vi "2ndStrikerPositionSkill.vi"(5 "Position":dbl[](array[numeric]), 7 "Time Elapsed?":bool=TRUE, 8 "error in (no error)":errorcluster, 9 "Game in":refnum<class "Game.lvclass">, 10 "Robot":refnum<class "Robot.lvclass">, 11 "2ndStrikerPositionSkill in":refnum<class "2ndStrikerPositionSkill.lvclass">) -> (0 "error out":errorcluster, 2 "2nd Striker Position":dbl[](array[numeric]), 3 "2ndStrikerPositionSkill out":refnum<class "2ndStrikerPositionSkill.lvclass">)   [LabVIEW 2018, in "2ndStrikerPositionSkill.lvclass"]
uses:
  2ndStrikerPositionSkill.lvclass
  Robot_class/Robot.lvclass
  C:/Users/Ronaldo/Desktop/Phoenix GIT/SSL_AI/Object_class/Object.lvclass
  Game_class/Game.lvclass
  Game_class/Game.lvclass/Game.ctl
  Referee_class/Referee.lvclass/Referee.ctl
  Team_class/Team.lvclass/Team.ctl
  Robot_class/Robot.lvclass/Robot.ctl
  Robot_class/roles.ctl
  Object_class/Object.lvclass/Object.ctl
  Utilities_class/Utilities.lvclass
  Object_class/Read x.vi
  Object_class/Read y.vi
  Robot_class/Read id.vi
  0c1a9825-39b9-4625-b9cc-4c6421953776.vi
  Team_class/Read RobotRef.vi
  7c6c6052-d6fd-4101-b52e-e5b07ba4cc6c.vi
  Referee_class/Read enemy_goalie_id.vi
  Game_class/Read EnemyRef.vi
  Game_class/Read AllyRef.vi
  Game_class/Read BallRef.vi
  Game_class/Read FieldRef.vi
  Game_class/Read Referee.vi
  Game_class/Read OffensiveTeam.vi
  <vilib>/Array/Sort 2D Array - Pop Stack.vi
  <vilib>/Array/Sort 2D Array - Push Stack.vi
  Ally_class/Ally.lvclass
  C:/Users/Ronaldo/Desktop/Phoenix GIT/SSL_AI/Team_class/Team.lvclass
  Enemy_class/Enemy.lvclass
  Ball_class/Ball.lvclass
  Field_class/Field.lvclass
  Referee_class/Referee.lvclass
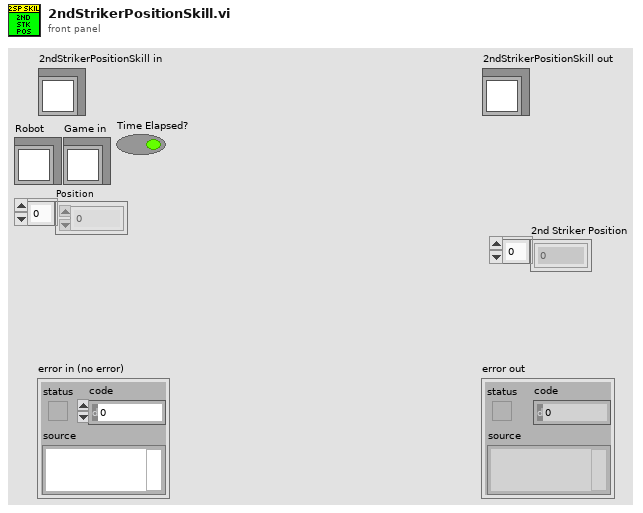
[diagram p1: front panel]
types:
  T1 = typedef "roles.ctl" = enum16{"PenaltyDefense", "PreparePassReceiver", "PassObserver", "Timeout", "Goto", "ZigZag", "None", "BallOutOfField", "DefenderArea", "Duelist", "AttackerStop", "FollowAttacker", "KeeperRole", "KickPenalty", "AttackerAimGoal", "AttackerBlock", "Marker", "Halt", "Shoot", "PassKicker", "PassReceiver", "TestRole", "PenaltyAttacker"}
  T2 = cluster{dbl[][], dbl, "Numeric":dbl, "Numeric":dbl}
  T3 = cluster{dbl[][], dbl, "Numeric":dbl, "Numeric":dbl, "I":dbl[]}
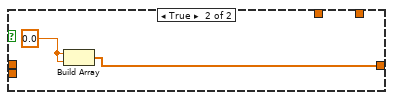
[diagram p3: hidden frame]
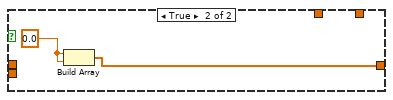
[diagram p4: hidden frame]
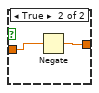
[diagram p5: hidden frame]
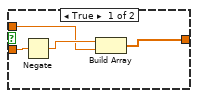
[diagram p9: hidden frame]
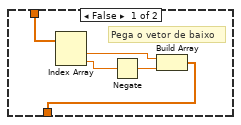
[diagram p10: hidden frame]
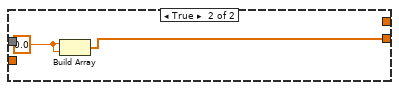
[diagram p12: hidden frame]
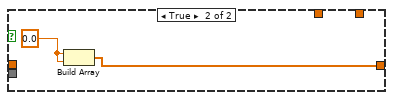
[diagram p13: hidden frame]
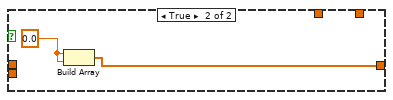
[diagram p17: hidden frame]
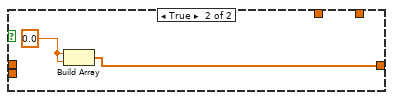
[diagram p18: hidden frame]
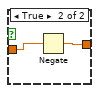
[diagram p19: hidden frame]
diagram:
  n1 = property class="Game"(reference="Game in") -> ("EnemyRef"=w7:refnum<class "Enemy.lvclass">, "AllyRef"=w4:refnum<class "Ally.lvclass">, "BallRef"=w5:refnum<class "Ball.lvclass">, "FieldRef"=w11:refnum<class "Field.lvclass">, "Referee"=w2:refnum<class "Referee.lvclass">, "OffensiveTeam"=w1:refnum<class "Ally.lvclass">)  [unwired: 1 in, 2 out]
  n2 = case shown="No Error" "error in (no error)" {
    selector: "error in (no error)" -> [w30 w734]
    tunnel: [w30 w734] -> w13
    tunnel: [w31 w733] -> w14
    tunnel: "2ndStrikerPositionSkill in" -> [w31 w733]
    tunnel: "Robot" -> [_ _]
    tunnel: w11 -> [w26 _]
    tunnel: w5 -> [_ _]
    tunnel: w7 -> [_ _]
    tunnel: w4 -> [_ _]
    tunnel: "Game in" -> [_ _]
    tunnel: "Time Elapsed?" -> [_ _]
    tunnel: "Position" -> [w29 _]
    tunnel: w7 -> [w25 _]
    tunnel: [w24 _] -> w6
    tunnel: w5 -> [w22 _]
    tunnel: "Robot" -> [w21 _]
    tunnel: w2 -> [w20 _]
    tunnel: w1 -> [w16 _]
    frame No Error {
      # "Verifica se y do 1st str é >= 0"
      n3 = property class="Referee"(reference=w20) -> ("enemy_goalie_id"=w19:i32)  [unwired: 1 in, 2 out]
      n4 = Index Array(array=w29) -> (element #2=w28:dbl)  [unwired: 2 in, 1 out]
      n5 = property class="Ally"(reference=w16) -> ("RobotRef"=w18:refnum<class "Robot.lvclass">[])  [unwired: 1 in, 2 out]
      n6 = Greater Or Equal?(x=w28, y=0.0 ("element")) -> (x >= y?=w23:bool)
      n7 = feedback-in #1(w18) -> ()
      n8 = feedback #1() -> (w17:refnum<class "Robot.lvclass">[])  [unwired: 1 in]
      n9 = case shown="True" w23 {
        tunnel: w26 -> [w137 w489]
        tunnel: w25 -> [w133 w485]
        tunnel: [w122 w474] -> w24
        tunnel: w22 -> [w126 w478]
        tunnel: w21 -> [w108 w460]
        tunnel: w19 -> [w119 w471]
        tunnel: w17 -> [w111 w463]
        frame True {
          w33 = refnum<class "Utilities.lvclass"> refnum ("Utilities in")
          w34 = refnum<class "Utilities.lvclass"> refnum ("Utilities in")
          w99 = refnum<class "Utilities.lvclass"> refnum ("Utilities in")
          (unwired) cluster{dbl[][], dbl, dbl, "y":dbl} {[], 0.0, 0.0, "y"=0.0}
          # "Novo Gap"
          # "Pegar o maior y, faz o mesmo, depois ve qual o maior gap desses 2"
          # "Angulo theta"
          # "Novo Gap"
          # "Pega o vetor de baixo"
          # "Pegar esse menor y, fazer o gap dele com o vetor de baixo e adicionar ao cluster"
          # "O menor y vai ser sempre menor que esse numero"
          # "Aqui entra o cluster"
          # "Tem que pegar os robos que estão nas extremidades, e ver o gap deles com os vetores das extremidades"
          # "Retorna o incentro aqui"
          # "Fazer outro for pra ver se o gap é o maior"
          # "Usar o primeiro elemento como inicial ao inves do zero -> evita erros"
          # "Se todos os robos adversários estão dentro do triangulo, passa as extremidades como robôs"
          # "(Field_length^2 + Field_width^2)^(1/2) / 4"
          # "Ver se a distancia do str é proxima da\ndo 2nd str"
          # "Achar a posição do striker"
          # "Ver se o 2nd striker ta perto do str"
          # "Se o robo esta a uma distância de 200mm da reta bola-gol"
          # "Fazer um if else caso o robo esteja muito proximo da reta do centro do gol ate a bola"
          # "Acha o incentro do triangulo"
          # "O if else evita que divida numero por zero\nSe o modulo do vetor for nulo, ele retorna o (0,0)"
          # "Soma com o vetor (L/2 , 0) pra achar os pontos que os vetores intersectam a reta"
          # "normaliza o vetor e multiplica por A"
          # "a = L/2 (senO/sen(O + O1))"
          # "Transforma os vetores em unitarios"
          # "Verifica quais robos estão na regiao delimitada"
          # "Calcula o ângulo fi (entre o eixo X e o ponto (L/3 , -h/2 -> no caso do triangulo em baixo)"
          # "pega o triangulo de baixo"
          n10 = property class="Enemy"(reference=w133) -> ("RobotRef"=w120:refnum<class "Robot.lvclass">[])  [unwired: 1 in, 2 out]
          n11 = call-dynamic "DeleteRobotByID.vi"("id"=w119, "RobotRef"=w120, "Utilities in"=refnum<class "Utilities.lvclass"> refnum) -> ("RobotRef out"=w118:refnum<class "Robot.lvclass">[])  [unwired: 6 in, 2 out]
          n12 = property class="Field"(reference=w137) -> ("field_length"=w101:i32, "field_width"=w102:i32)  [unwired: 1 in, 2 out]
          n13 = Divide(x=w101, y=6) -> (x/y=w116:dbl)
          n14 = Multiply(x=w116, y=1) -> (x*y=w114:dbl)
          n15 = Divide(x=w101, y=2) -> (x/y=w65:dbl)
          n16 = Divide(x=w102, y=2) -> (x/y=w129:dbl)
          n17 = Build Array(w65, 0.0 ("element")) -> (w44:dbl[])
          n18 = for {
            tunnel: w118 -> [w383] mode=indexing
            tunnel: w44 -> [w377]
            tunnel: [w381] -> w93 mode=indexing if=w372
            # "Só vai considerar os robos dentro da regiao, com y<0 e x>0 (depois do meio campo)"
            # "Trabalhar com os angulos em modulo, e ver se o y é menor que zero"
            n19 = property class="Robot"(reference=w383) -> ("x"=w373:dbl, "y"=w378:dbl, "id"=w371:i32)  [unwired: 1 in, 2 out]
            n20 = Build Array(w373, w378) -> (w382:dbl[])
            n21 = Subtract(x=w382, y=w377) -> (x-y=w380:dbl[])
            n22 = Negate(x=w377) -> (-x=w376:dbl[])
            n23 = call "AngleBetween2Vectors.vi"("Array 1"=w376, "Array 2"=w380, "Utilities in"=refnum<class "Utilities.lvclass"> refnum) -> ("Numeric"=w375:dbl)  [unwired: 6 in, 2 out]
            n24 = Build Array (concatenate)(w380, w375, w371) -> (w381:dbl[])
            n25 = Greater?(x=w373, y=0.0) -> (0:w372:bool)
          }
          n26 = Build Array(w114, w129) -> (w113:dbl[])
          n27 = Build Array(w102, w101) -> (w100:i32[])
          n28 = Subtract(x=w113, y=w44) -> (x-y=w43:dbl[])
          n29 = Negate(x=w44) -> (-x=w127:dbl[])
          n30 = call-dynamic "Module.vi"("2D vector"=w100, "Utilities in"=w99) -> ("Modulo"=w98:dbl)  [unwired: 7 in, 2 out]
          n31 = call "AngleBetween2Vectors.vi"("Array 1"=w127, "Array 2"=w43, "Utilities in"=w99) -> ("Numeric"=w87:dbl)  [unwired: 6 in, 2 out]
          n32 = for {
            tunnel: w93 -> [w195] mode=indexing
            tunnel: w87 -> [w193]
            shift-right: [w190] -> w94
            shift-left: TRUE -> [w191]
            (unwired) TRUE
            n33 = Index Array(array=w195) -> (element #3=w194:dbl)  [unwired: 3 in, 2 out]
            n34 = Less Or Equal?(x=w194, y=w193) -> (x <= y?=w192:bool)
            n35 = And(x=w191, y=w192) -> (x .and. y?=w190:bool)
          }
          n36 = case shown="True" w94 {
            tunnel: w93 -> [w196 w208]
            tunnel: [w196 w207] -> w92
            tunnel: w43 -> [_ w205]
            tunnel: w87 -> [_ w199]
            frame False {
            }
            frame True {
              # "Adiciona os vetores das extremidades"
              n37 = Index Array(array=w205) -> (element #1=w204:dbl, element #2=w203:dbl)  [unwired: 2 in]
              n38 = Build Array (concatenate)(w205, w199, 10) -> (w201:dbl[])
              n39 = Negate(x=w203) -> (-x=w202:dbl)
              n40 = Build Array(w204, w202) -> (w200:dbl[])
              n41 = Build Array (concatenate)(w200, w199, 11) -> (w197:dbl[])
              n42 = Insert Into Array(array=w208, new element #1=w201, new element #2=w197) -> (w207:dbl[][])  [unwired: 2 in]
            }
          }
          n43 = call "Sort 2D Array.vim"("index"=1, "dimension to index (column)"=enum16{"column", "row"}."column", "2D array"=w92) -> ("sorted 2D array"=w91:dbl[][])  [unwired: 7 in, 1 out]
          n44 = Index Array(array=w91) -> (element #1=w90:dbl[])  [unwired: 4 in, 1 out]
          n45 = Index Array(array=w90) -> (element #1=w89:dbl, element #2=w82:dbl, element #3=w80:dbl)  [unwired: 4 in, 1 out]
          n46 = Less?(x=w82, y=0.0) -> (x < y?=w81:bool)
          n47 = case shown="False" w81 {
            tunnel: [w179 w181] -> w79
            tunnel: w80 -> [w179 w180]
            frame False {
            }
            frame True {
              n48 = Negate(x=w180) -> (-x=w181:dbl)
            }
          }
          n49 = Build Array(w89, w82) -> (w88:dbl[])
          n50 = for {
            tunnel: w91 -> [w367] mode=indexing
            shift-right: [w354] -> _
            shift-left: w79 -> [w361]
            shift-right: [w365] -> _
            shift-left: w88 -> [w364]
            tunnel: [w362] -> w128 mode=indexing
            # "Pega o modulo pro caso do 0 e de um angulo neg"
            # "Se o y é negativo, faz o angulo ser negativo\npra quando fazer a difrença de um positivo com um neg\nele somar"
            # "Faz a diferença entre os angulos pra achar os gaps"
            n51 = Index Array(array=w367) -> (element #1=w366:dbl, element #2=w356:dbl, element #3=w355:dbl)  [unwired: 3 in]
            n52 = Less?(x=w356, y=0.0) -> (x < y?=w358:bool)
            n53 = case shown="True" w358 {
              tunnel: w355 -> [w368 w370]
              tunnel: [w368 w369] -> w354
              frame False {
              }
              frame True {
                n54 = Negate(x=w370) -> (-x=w369:dbl)
              }
            }
            n55 = Subtract(x=w354, y=w361) -> (x-y=w360:dbl)
            n56 = Absolute Value(x=w360) -> (abs(x)=w359:dbl)
            n57 = Build Array(w366, w356) -> (w365:dbl[])
            n58 = Build Array(w365, w364) -> (w363:dbl[][])
            n59 = Bundle(w363, w359, "Numeric"=w354, "Numeric"=w361) -> (w362:T2)  [unwired: 1 in]
          }
          n60 = for {
            tunnel: w128 -> [w277] mode=indexing
            tunnel: w87 -> [w276]
            tunnel: w44 -> [w295]
            tunnel: w113 -> [w294]
            tunnel: w65 -> [w290]
            tunnel: w44 -> [w283]
            tunnel: w44 -> [w280]
            tunnel: [w255] -> w112
            tunnel: w44 -> [w258]
            tunnel: w44 -> [w274]
            tunnel: w43 -> [w257]
            tunnel: w87 -> [w256]
            tunnel: [w254] -> w56 mode=indexing if=w245
            tunnel: [w250] -> w52
            w255 = refnum<class "Utilities.lvclass"> refnum ("Utilities in")
            w299 = refnum<class "Utilities.lvclass"> refnum ("Utilities in")
            # "Só vai passar aqueles que a bissetriz ta dentro do traingulo"
            # "E o gap é diferente de zeo\npra poder tirar o primeiro elemento"
            # "Se der false, tem que calcular o incentro novo, e o gap novo"
            # "no novo cluster vai ter tudo do antigo, mais o incentro"
            # "Se o incentro esta dentro do triangulo\npassa o incentro certo"
            # "Angulo theta"
            # "Retorna o gap e os vetores que formam o gap"
            # "Ve qual o maior gap"
            n61 = Unbundle(w277) -> (w265:dbl[][], w249:dbl, "Numeric"=w262:dbl, "Numeric"=w261:dbl)
            n62 = Unbundle(w277) -> (w302:dbl[][], "Numeric"=w269:dbl, "Numeric"=w271:dbl)  [unwired: 1 out]
            n63 = Absolute Value(x=w271) -> (abs(x)=w270:dbl)
            n64 = Absolute Value(x=w269) -> (abs(x)=w268:dbl)
            n65 = Index Array(array=w302) -> (element #1=w301:dbl[], element #2=w300:dbl[])  [unwired: 4 in]
            n66 = call-dynamic "Module.vi"("2D vector"=w300, "Utilities in"=w299) -> ("Modulo"=w297:dbl)  [unwired: 7 in, 2 out]
            n67 = call-dynamic "Module.vi"("2D vector"=w301, "Utilities in"=w299) -> ("Modulo"=w298:dbl)  [unwired: 7 in, 2 out]
            n68 = call "AngleBetween2Vectors.vi"("Array 1"=w295, "Array 2"=w294, "Utilities in"=refnum<class "Utilities.lvclass"> refnum) -> ("Numeric"=w250:dbl)  [unwired: 6 in, 2 out]
            n69 = Equal?(x=w298, y=0) -> (x = y?=w285:bool)
            n70 = Add(x=w250, y=w270) -> (x+y=w291:dbl)
            n71 = Add(x=w250, y=w268) -> (x+y=w292:dbl)
            n72 = Sine(x=w250) -> (sin(x)=w289:dbl)
            n73 = Sine(x=w292) -> (sin(x)=w287:dbl)
            n74 = Sine(x=w291) -> (sin(x)=w286:dbl)
            n75 = Equal?(x=w297, y=0) -> (x = y?=w281:bool)
            n76 = Multiply(x=w289, y=w290) -> (x*y=w288:dbl)
            n77 = Divide(x=w288, y=w287) -> (x/y=w284:dbl)
            n78 = case shown="False" w285 {
              tunnel: w301 -> [w351 _]
              tunnel: w298 -> [w350 _]
              tunnel: w284 -> [w349 _]
              tunnel: w283 -> [w346 _]
              tunnel: [w345 w352] -> w278
              frame False {
                n79 = Divide(x=w351, y=w350) -> (x/y=w348:dbl[])
                n80 = Multiply(x=w348, y=w349) -> (x*y=w347:dbl[])
                n81 = Add(x=w346, y=w347) -> (x+y=w345:dbl[])
              }
              frame True {
                w353 = 0.0
                n82 = Build Array(w353, w353) -> (w352:dbl[])
              }
            }
            n83 = Divide(x=w288, y=w286) -> (x/y=w253:dbl)
            n84 = case shown="False" w281 {
              tunnel: w300 -> [w342 _]
              tunnel: w297 -> [w336 _]
              tunnel: w253 -> [w341 _]
              tunnel: w280 -> [w337 _]
              tunnel: [w338 w343] -> w279
              tunnel: [w337 _] -> w252
              tunnel: [w336 _] -> w251
              frame False {
                n85 = Divide(x=w342, y=w336) -> (x/y=w340:dbl[])
                n86 = Multiply(x=w340, y=w341) -> (x*y=w339:dbl[])
                n87 = Add(x=w337, y=w339) -> (x+y=w338:dbl[])
              }
              frame True {
                w344 = 0.0
                n88 = Build Array(w344, w344) -> (w343:dbl[])
              }
            }
            n89 = call "IncenterTriangle.vi"("C"=w279, "B"=w278, "A"=w258, "Utilities in"=w255) -> ("I"=w267:dbl[])  [unwired: 5 in, 2 out]
            n90 = Subtract(x=w267, y=w274) -> (x-y=w275:dbl[])
            n91 = Negate(x=w274) -> (-x=w273:dbl[])
            n92 = call "AngleBetween2Vectors.vi"("Array 1"=w273, "Array 2"=w275, "Utilities in"=w255) -> ("Numeric"=w272:dbl)  [unwired: 6 in, 2 out]
            n93 = Equal?(x=0.0, y=w249) -> (x = y?=w247:bool)
            n94 = Less Or Equal?(x=w272, y=w276) -> (x <= y?=w245:bool)
            n95 = Or(x=w245, y=w247) -> (x .or. y?=w246:bool)
            n96 = case shown="False" w246 {
              tunnel: w267 -> [_ w335]
              tunnel: [w319 w335] -> w266
              tunnel: w265 -> [w324 w334]
              tunnel: [w317 w334] -> w264
              tunnel: w249 -> [_ w333]
              tunnel: [w313 w333] -> w263
              tunnel: w262 -> [_ w332]
              tunnel: w261 -> [w315 w331]
              tunnel: [w316 w332] -> w260
              tunnel: [w315 w331] -> w259
              tunnel: w258 -> [w323 _]
              tunnel: w257 -> [w320 _]
              tunnel: w256 -> [w316 _]
              tunnel: w255 -> [w312 _]
              tunnel: w253 -> [w307 _]
              tunnel: w252 -> [w306 _]
              tunnel: w251 -> [w304 _]
              frame False {
                # "Tem que fazer isso pra colocar o ponto na posição correta e em relação ao centro do campo"
                # "Novo Gap"
                # "Se o os vetores estiverem abaixo do meio campo\npega o veotr pra baixo\nSe estiverem acima, pega o voter de cima"
                n97 = Index Array(array=w324) -> (element #1=w322:dbl[], element #2=w303:dbl[])  [unwired: 4 in]
                n98 = Index Array(array=w322) -> (element #2=w311:dbl)  [unwired: 2 in, 1 out]
                n99 = Greater?(x=w311, y=0.0) -> (0:w321:bool)
                n100 = Divide(x=w303, y=w304) -> (x/y=w309:dbl[])
                n101 = Multiply(x=w309, y=w307) -> (x*y=w308:dbl[])
                n102 = case shown="True" w321 {
                  tunnel: w320 -> [w329 w330]
                  tunnel: [w325 w330] -> w318
                  frame False {
                    # "Pega o vetor de baixo"
                    n103 = Index Array(array=w329) -> (element #1=w326:dbl, element #2=w328:dbl)  [unwired: 2 in]
                    n104 = Negate(x=w328) -> (-x=w327:dbl)
                    n105 = Build Array(w326, w327) -> (w325:dbl[])
                  }
                  frame True {
                  }
                }
                n106 = Add(x=w306, y=w308) -> (x+y=w305:dbl[])
                n107 = call "IncenterTriangle.vi"("C"=w305, "B"=w323, "A"=w318, "Utilities in"=w312) -> ("I"=w319:dbl[])  [unwired: 5 in, 2 out]
                n108 = Build Array(w318, w303) -> (w317:dbl[][])
                n109 = Subtract(x=w316, y=w315) -> (x-y=w314:dbl)
                n110 = Absolute Value(x=w314) -> (abs(x)=w313:dbl)
              }
              frame True {
              }
            }
            n111 = Bundle(w264, w263, "Numeric"=w260, "Numeric"=w259, "I"=w266) -> (w254:T3)  [unwired: 1 in]
          }
          n112 = for {
            tunnel: w56 -> [w178] mode=indexing
            shift-right: [w176] -> _
            shift-left: 10000.0 ("Numeric") -> [w175]
            shift-right: [w173] -> _
            shift-left: -10000.0 ("Numeric") -> [w172]
            shift-right: [w171] -> w62
            shift-left: dbl[] [] -> [w170]
            shift-right: [w168] -> w48
            shift-left: dbl[] [] -> [w167]
            shift-right: [w165] -> w67
            shift-left: 0.0 ("Numeric") -> [w164]
            shift-right: [w161] -> w53
            shift-left: 0.0 ("Numeric") -> [w160]
            # "Pegar aqui o maior y"
            # "Pegar aqui o menor y"
            n113 = Unbundle(w178) -> (w177:dbl[][], "Numeric"=w163:dbl)  [unwired: 3 out]
            n114 = Index Array(array=w177) -> (element #2=w169:dbl[])  [unwired: 4 in, 1 out]
            n115 = Index Array(array=w169) -> (element #2=w174:dbl)  [unwired: 2 in, 1 out]
            n116 = Less?(x=w174, y=w175) -> (x < y?=w166:bool)
            n117 = Greater?(x=w174, y=w172) -> (0:w162:bool)
            n118 = Select(t=w174, s=w166, f=w175) -> (s? t:f=w176:dbl)
            n119 = Select(t=w169, s=w166, f=w170) -> (s? t:f=w171:dbl[])
            n120 = Select(t=w163, s=w166, f=w164) -> (s? t:f=w165:dbl)
            n121 = Select(t=w163, s=w162, f=w160) -> (s? t:f=w161:dbl)
            n122 = Select(t=w169, s=w162, f=w167) -> (s? t:f=w168:dbl[])
            n123 = Select(t=w174, s=w162, f=w172) -> (s? t:f=w173:dbl)
          }
          n124 = Index Array(array=w43) -> (element #1=w70:dbl, element #2=w72:dbl)  [unwired: 2 in]
          n125 = Negate(x=w72) -> (-x=w71:dbl)
          n126 = Build Array(w70, w71) -> (w58:dbl[])
          n127 = Add(x=w52, y=w67) -> (x+y=w66:dbl)
          n128 = Add(x=w52, y=w53) -> (x+y=w51:dbl)
          n129 = call-dynamic "Module.vi"("2D vector"=w48, "Utilities in"=w33) -> ("Modulo"=w47:dbl)  [unwired: 7 in, 2 out]
          n130 = call-dynamic "Module.vi"("2D vector"=w62, "Utilities in"=w34) -> ("Modulo"=w61:dbl)  [unwired: 7 in, 2 out]
          n131 = Sine(x=w52) -> (sin(x)=w64:dbl)
          n132 = Sine(x=w51) -> (sin(x)=w50:dbl)
          n133 = Sine(x=w66) -> (sin(x)=w63:dbl)
          n134 = call "AngleBetween2Vectors.vi"("Array 1"=w48, "Array 2"=w43, "Utilities in"=w33) -> ("Numeric"=w35:dbl)  [unwired: 6 in, 2 out]
          n135 = Equal?(x=w61, y=0) -> (x = y?=w68:bool)
          n136 = call "AngleBetween2Vectors.vi"("Array 1"=w62, "Array 2"=w58, "Utilities in"=w34) -> ("Numeric"=w38:dbl)  [unwired: 6 in, 2 out]
          n137 = Multiply(x=w65, y=w64) -> (x*y=w49:dbl)
          n138 = Divide(x=w49, y=w50) -> (x/y=w46:dbl)
          n139 = Equal?(x=w47, y=0) -> (x = y?=w54:bool)
          n140 = Divide(x=w49, y=w63) -> (x/y=w60:dbl)
          n141 = case shown="False" w68 {
            tunnel: w62 -> [w157 _]
            tunnel: w61 -> [w156 _]
            tunnel: w60 -> [w155 _]
            tunnel: w44 -> [w152 _]
            tunnel: [w151 w158] -> w59
            frame False {
              n142 = Divide(x=w157, y=w156) -> (x/y=w154:dbl[])
              n143 = Multiply(x=w154, y=w155) -> (x*y=w153:dbl[])
              n144 = Add(x=w152, y=w153) -> (x+y=w151:dbl[])
            }
            frame True {
              w159 = 0.0
              n145 = Build Array(w159, w159) -> (w158:dbl[])
            }
          }
          n146 = case shown="False" w54 {
            tunnel: w47 -> [w143 _]
            tunnel: w48 -> [w142 _]
            tunnel: w46 -> [w148 _]
            tunnel: w44 -> [w145 _]
            tunnel: [w144 w149] -> w45
            frame False {
              n147 = Divide(x=w142, y=w143) -> (x/y=w147:dbl[])
              n148 = Multiply(x=w147, y=w148) -> (x*y=w146:dbl[])
              n149 = Add(x=w145, y=w146) -> (x+y=w144:dbl[])
            }
            frame True {
              w150 = 0.0
              n150 = Build Array(w150, w150) -> (w149:dbl[])
            }
          }
          n151 = Add(x=w58, y=w44) -> (x+y=w57:dbl[])
          n152 = Add(x=w44, y=w43) -> (x+y=w42:dbl[])
          n153 = call "IncenterTriangle.vi"("C"=w44, "B"=w59, "A"=w57, "Utilities in"=w34) -> ("I"=w40:dbl[])  [unwired: 5 in, 2 out]
          n154 = call "IncenterTriangle.vi"("C"=w42, "B"=w44, "A"=w45, "Utilities in"=w34) -> ("I"=w36:dbl[])  [unwired: 5 in, 2 out]
          n155 = Greater?(x=w38, y=w35) -> (0:w41:bool)
          n156 = case shown="False" w41 {
            tunnel: w40 -> [_ w141]
            tunnel: [w139 w141] -> w39
            tunnel: w38 -> [_ w140]
            tunnel: [w138 w140] -> w37
            tunnel: w36 -> [w139 _]
            tunnel: w35 -> [w138 _]
            frame False {
            }
            frame True {
            }
          }
          n157 = for {
            tunnel: w56 -> [w189] mode=indexing
            shift-right: [w188] -> _
            shift-left: w37 -> [w182]
            shift-right: [w186] -> w86
            shift-left: w39 -> [w185]
            # "Vai retornar o incentro"
            n158 = Unbundle(w189) -> (w183:dbl, "I"=w187:dbl[])  [unwired: 3 out]
            n159 = Less?(x=w182, y=w183) -> (x < y?=w184:bool)
            n160 = Select(t=w187, s=w184, f=w185) -> (s? t:f=w186:dbl[])
            n161 = Select(t=w183, s=w184, f=w182) -> (s? t:f=w188:dbl)
          }
          n162 = call "FindRobotByRole.vi"("role"=roles."PreparePassReceiver", "RobotRef"=w111, "Utilities in"=w112) -> ("Robots"=w109:refnum<class "Robot.lvclass">[])  [unwired: 6 in, 2 out]
          n163 = property class="Robot"(reference=w108) -> ("id"=w107:i32)  [unwired: 1 in, 2 out]
          n164 = for {
            tunnel: w109 -> [w213] mode=indexing
            tunnel: w107 -> [w214]
            tunnel: [w210] -> w106 mode=indexing if=w209
            n165 = property class="Robot"(reference=w213) -> ("id"=w215:i32, "x"=w212:dbl, "y"=w211:dbl)  [unwired: 1 in, 2 out]
            n166 = Not Equal?(x=w215, y=w214) -> (x != y?=w209:bool)
            n167 = Build Array(w212, w211) -> (w210:dbl[])
          }
          n168 = Index Array(array=w106) -> (element=w105:dbl[])  [unwired: 2 in]
          n169 = call-dynamic "Distance.vi"("P1"=w86, "P2"=w105, "Utilities in"=w112) -> ("Distance"=w104:dbl)  [unwired: 6 in, 2 out]
          n170 = Divide(x=w98, y=10.0) -> (x/y=w96:dbl)
          n171 = Less?(x=w104, y=w96) -> (x < y?=w32:bool)
          n172 = case shown="True" w32 {
            tunnel: [w216 w218] -> w85
            tunnel: w86 -> [w216 w217]
            frame False {
              # "Se der falso, pasa a posição calculada anteriormente"
            }
            frame True {
              # "se der true, ele se move em direção ao centro do campo"
              n173 = Multiply(x=w217, y=0.6) -> (x*y=w218:dbl[])
            }
          }
          n174 = property class="Ball"(reference=w126) -> ("x"=w125:dbl, "y"=w103:dbl)  [unwired: 1 in, 2 out]
          n175 = Build Array(w125, w103) -> (w121:dbl[])
          n176 = call-dynamic "DistancePointLine.vi"("Q"=w85, "P2"=w121, "P1"=w44, "Utilities in"=w112) -> ("distance"=w124:dbl)  [unwired: 5 in, 2 out]
          n177 = Less Or Equal?(x=w124, y=250.0) -> (x <= y?=w84:bool)
          n178 = case shown="True" w84 {
            tunnel: [w220 w228] -> w122
            tunnel: w121 -> [_ w236]
            tunnel: w44 -> [_ w235]
            tunnel: w103 -> [_ w224]
            tunnel: w85 -> [w220 w221]
            frame False {
            }
            frame True {
              # "Se ybola>0, pega o vetor (-b,a) caso contrario, pega o (b,-a)"
              # "Soma com o vetor x pra fazer em relação ao centro do  campo"
              # "normaliza ele"
              # "(a,b) o perpendicular em direção\n ao entro do campo é (-b,a)\nbola na parte de cima"
              # "Vetor bola-gol"
              # "Ele se move na perpendicular em relação à reta bola gol\nem direção ao meio do campo"
              # "Distância do robo ate a linha da bola-gol"
              n179 = Subtract(x=w236, y=w235) -> (x-y=w234:dbl[])
              n180 = Index Array(array=w234) -> (element #1=w226:dbl, element #2=w227:dbl)  [unwired: 2 in]
              n181 = Greater?(x=w224, y=0.0) -> (0:w222:bool)
              n182 = case shown="False" w222 {
                tunnel: w227 -> [w240 w241]
                tunnel: w226 -> [w238 w243]
                tunnel: [w237 w244] -> w225
                frame True {
                  n183 = Negate(x=w240) -> (-x=w239:dbl)
                  n184 = Build Array(w239, w238) -> (w237:dbl[])
                }
                frame False {
                  n185 = Negate(x=w243) -> (-x=w242:dbl)
                  n186 = Build Array(w241, w242) -> (w244:dbl[])
                }
              }
              n187 = call-dynamic "Module.vi"("2D vector"=w225, "Utilities in"=refnum<class "Utilities.lvclass"> refnum) -> ("Modulo"=w232:dbl)  [unwired: 7 in, 2 out]
              n188 = Divide(x=w225, y=w232) -> (x/y=w231:dbl[])
              n189 = Multiply(x=600.0, y=w231) -> (x*y=w229:dbl[])
              n190 = Add(x=w221, y=w229) -> (x+y=w228:dbl[])
            }
          }
        }
        frame False {
          w384 = refnum<class "Utilities.lvclass"> refnum ("Utilities in")
          w385 = refnum<class "Utilities.lvclass"> refnum ("Utilities in")
          w450 = refnum<class "Utilities.lvclass"> refnum ("Utilities in")
          (unwired) cluster{dbl[][], dbl, dbl, "y":dbl} {[], 0.0, 0.0, "y"=0.0}
          # "Novo Gap"
          # "Pegar o maior y, faz o mesmo, depois ve qual o maior gap desses 2"
          # "Angulo theta"
          # "Novo Gap"
          # "Pega o vetor de baixo"
          # "Pegar esse menor y, fazer o gap dele com o vetor de baixo e adicionar ao cluster"
          # "O menor y vai ser sempre menor que esse numero"
          # "Aqui entra o cluster"
          # "Tem que pegar os robos que estão nas extremidades, e ver o gap deles com os vetores das extremidades"
          # "Retorna o incentro aqui"
          # "Fazer outro for pra ver se o gap é o maior"
          # "Usar o primeiro elemento como inicial ao inves do zero -> evita erros"
          # "Se todos os robos adversários estão dentro do triangulo, passa as extremidades como robôs"
          # "(Field_length^2 + Field_width^2)^(1/2) / 4"
          # "Ver se a distancia do str é proxima da\ndo 2nd str"
          # "Achar a posição do striker"
          # "Ver se o 2nd striker ta perto do str"
          # "Se o robo esta a uma distância de 200mm da reta bola-gol"
          # "Fazer um if else caso o robo esteja muito proximo da reta do centro do gol ate a bola"
          # "Acha o incentro do triangulo"
          # "O if else evita que divida numero por zero\nSe o modulo do vetor for nulo, ele retorna o (0,0)"
          # "Soma com o vetor (L/2 , 0) pra achar os pontos que os vetores intersectam a reta"
          # "normaliza o vetor e multiplica por A"
          # "a = L/2 (senO/sen(O + O1))"
          # "Transforma os vetores em unitarios"
          # "Verifica quais robos estão na regiao delimitada"
          # "Calcula o ângulo fi (entre o eixo X e o ponto (L/3 , -h/2 -> no caso do triangulo em baixo)"
          # "pega o triangulo de baixo"
          n191 = property class="Enemy"(reference=w485) -> ("RobotRef"=w472:refnum<class "Robot.lvclass">[])  [unwired: 1 in, 2 out]
          n192 = call-dynamic "DeleteRobotByID.vi"("id"=w471, "RobotRef"=w472, "Utilities in"=refnum<class "Utilities.lvclass"> refnum) -> ("RobotRef out"=w470:refnum<class "Robot.lvclass">[])  [unwired: 6 in, 2 out]
          n193 = property class="Field"(reference=w489) -> ("field_length"=w452:i32, "field_width"=w453:i32)  [unwired: 1 in, 2 out]
          n194 = Divide(x=w452, y=6) -> (x/y=w468:dbl)
          n195 = Multiply(x=w468, y=1) -> (x*y=w466:dbl)
          n196 = Divide(x=w452, y=2) -> (x/y=w416:dbl)
          n197 = Divide(x=w453, y=-2) -> (x/y=w481:dbl)
          n198 = Build Array(w416, 0.0 ("element")) -> (w395:dbl[])
          n199 = for {
            tunnel: w470 -> [w732] mode=indexing
            tunnel: w395 -> [w726]
            tunnel: [w730] -> w444 mode=indexing if=w721
            # "Só vai considerar os robos dentro da regiao, com y<0 e x>0 (depois do meio campo)"
            # "Trabalhar com os angulos em modulo, e ver se o y é menor que zero"
            n200 = property class="Robot"(reference=w732) -> ("x"=w722:dbl, "y"=w727:dbl, "id"=w720:i32)  [unwired: 1 in, 2 out]
            n201 = Build Array(w722, w727) -> (w731:dbl[])
            n202 = Subtract(x=w731, y=w726) -> (x-y=w729:dbl[])
            n203 = Negate(x=w726) -> (-x=w725:dbl[])
            n204 = call "AngleBetween2Vectors.vi"("Array 1"=w725, "Array 2"=w729, "Utilities in"=refnum<class "Utilities.lvclass"> refnum) -> ("Numeric"=w724:dbl)  [unwired: 6 in, 2 out]
            n205 = Build Array (concatenate)(w729, w724, w720) -> (w730:dbl[])
            n206 = Greater?(x=w722, y=0.0) -> (0:w721:bool)
          }
          n207 = Build Array(w466, w481) -> (w465:dbl[])
          n208 = Build Array(w453, w452) -> (w451:i32[])
          n209 = Subtract(x=w465, y=w395) -> (x-y=w394:dbl[])
          n210 = Negate(x=w395) -> (-x=w479:dbl[])
          n211 = call-dynamic "Module.vi"("2D vector"=w451, "Utilities in"=w450) -> ("Modulo"=w449:dbl)  [unwired: 7 in, 2 out]
          n212 = call "AngleBetween2Vectors.vi"("Array 1"=w479, "Array 2"=w394, "Utilities in"=w450) -> ("Numeric"=w438:dbl)  [unwired: 6 in, 2 out]
          n213 = for {
            tunnel: w444 -> [w547] mode=indexing
            tunnel: w438 -> [w545]
            shift-right: [w542] -> w445
            shift-left: TRUE -> [w543]
            (unwired) TRUE
            n214 = Index Array(array=w547) -> (element #3=w546:dbl)  [unwired: 3 in, 2 out]
            n215 = Less Or Equal?(x=w546, y=w545) -> (x <= y?=w544:bool)
            n216 = And(x=w543, y=w544) -> (x .and. y?=w542:bool)
          }
          n217 = case shown="True" w445 {
            tunnel: w444 -> [w548 w560]
            tunnel: [w548 w559] -> w443
            tunnel: w394 -> [_ w557]
            tunnel: w438 -> [_ w551]
            frame False {
            }
            frame True {
              # "Adiciona os vetores das extremidades"
              n218 = Index Array(array=w557) -> (element #1=w556:dbl, element #2=w555:dbl)  [unwired: 2 in]
              n219 = Build Array (concatenate)(w557, w551, 10) -> (w553:dbl[])
              n220 = Negate(x=w555) -> (-x=w554:dbl)
              n221 = Build Array(w556, w554) -> (w552:dbl[])
              n222 = Build Array (concatenate)(w552, w551, 11) -> (w549:dbl[])
              n223 = Insert Into Array(array=w560, new element #1=w553, new element #2=w549) -> (w559:dbl[][])  [unwired: 2 in]
            }
          }
          n224 = call "Sort 2D Array.vim"("index"=1, "dimension to index (column)"=enum16{"column", "row"}."column", "2D array"=w443) -> ("sorted 2D array"=w442:dbl[][])  [unwired: 7 in, 1 out]
          n225 = Index Array(array=w442) -> (element #1=w441:dbl[])  [unwired: 4 in, 1 out]
          n226 = Index Array(array=w441) -> (element #1=w440:dbl, element #2=w433:dbl, element #3=w431:dbl)  [unwired: 4 in, 1 out]
          n227 = Less?(x=w433, y=0.0) -> (x < y?=w432:bool)
          n228 = case shown="False" w432 {
            tunnel: [w531 w533] -> w430
            tunnel: w431 -> [w531 w532]
            frame False {
            }
            frame True {
              n229 = Negate(x=w532) -> (-x=w533:dbl)
            }
          }
          n230 = Build Array(w440, w433) -> (w439:dbl[])
          n231 = for {
            tunnel: w442 -> [w716] mode=indexing
            shift-right: [w703] -> _
            shift-left: w430 -> [w710]
            shift-right: [w714] -> _
            shift-left: w439 -> [w713]
            tunnel: [w711] -> w480 mode=indexing
            # "Pega o modulo pro caso do 0 e de um angulo neg"
            # "Se o y é negativo, faz o angulo ser negativo\npra quando fazer a difrença de um positivo com um neg\nele somar"
            # "Faz a diferença entre os angulos pra achar os gaps"
            n232 = Index Array(array=w716) -> (element #1=w715:dbl, element #2=w705:dbl, element #3=w704:dbl)  [unwired: 3 in]
            n233 = Less?(x=w705, y=0.0) -> (x < y?=w707:bool)
            n234 = case shown="True" w707 {
              tunnel: w704 -> [w717 w719]
              tunnel: [w717 w718] -> w703
              frame False {
              }
              frame True {
                n235 = Negate(x=w719) -> (-x=w718:dbl)
              }
            }
            n236 = Subtract(x=w703, y=w710) -> (x-y=w709:dbl)
            n237 = Absolute Value(x=w709) -> (abs(x)=w708:dbl)
            n238 = Build Array(w715, w705) -> (w714:dbl[])
            n239 = Build Array(w714, w713) -> (w712:dbl[][])
            n240 = Bundle(w712, w708, "Numeric"=w703, "Numeric"=w710) -> (w711:T2)  [unwired: 1 in]
          }
          n241 = for {
            tunnel: w480 -> [w626] mode=indexing
            tunnel: w438 -> [w625]
            tunnel: w395 -> [w644]
            tunnel: w465 -> [w643]
            tunnel: w416 -> [w639]
            tunnel: w395 -> [w632]
            tunnel: w395 -> [w629]
            tunnel: [w602] -> w464
            tunnel: w395 -> [w605]
            tunnel: w395 -> [w623]
            tunnel: w394 -> [w604]
            tunnel: w438 -> [w603]
            tunnel: [w601] -> w407 mode=indexing
            tunnel: [w597] -> w403
            w602 = refnum<class "Utilities.lvclass"> refnum ("Utilities in")
            w648 = refnum<class "Utilities.lvclass"> refnum ("Utilities in")
            # "Se der false, tem que calcular o incentro novo, e o gap novo"
            # "no novo cluster vai ter tudo do antigo, mais o incentro"
            # "Se o incentro esta dentro do triangulo\npassa o incentro certo"
            # "Angulo theta"
            # "Retorna o gap e os vetores que formam o gap"
            # "Ve qual o maior gap"
            n242 = Unbundle(w626) -> (w613:dbl[][], w611:dbl, "Numeric"=w609:dbl, "Numeric"=w608:dbl)
            n243 = Unbundle(w626) -> (w651:dbl[][], "Numeric"=w618:dbl, "Numeric"=w620:dbl)  [unwired: 1 out]
            n244 = Absolute Value(x=w620) -> (abs(x)=w619:dbl)
            n245 = Absolute Value(x=w618) -> (abs(x)=w617:dbl)
            n246 = Index Array(array=w651) -> (element #1=w650:dbl[], element #2=w649:dbl[])  [unwired: 4 in]
            n247 = call-dynamic "Module.vi"("2D vector"=w649, "Utilities in"=w648) -> ("Modulo"=w646:dbl)  [unwired: 7 in, 2 out]
            n248 = call-dynamic "Module.vi"("2D vector"=w650, "Utilities in"=w648) -> ("Modulo"=w647:dbl)  [unwired: 7 in, 2 out]
            n249 = call "AngleBetween2Vectors.vi"("Array 1"=w644, "Array 2"=w643, "Utilities in"=refnum<class "Utilities.lvclass"> refnum) -> ("Numeric"=w597:dbl)  [unwired: 6 in, 2 out]
            n250 = Equal?(x=w647, y=0) -> (x = y?=w634:bool)
            n251 = Add(x=w597, y=w619) -> (x+y=w640:dbl)
            n252 = Add(x=w597, y=w617) -> (x+y=w641:dbl)
            n253 = Sine(x=w597) -> (sin(x)=w638:dbl)
            n254 = Sine(x=w641) -> (sin(x)=w636:dbl)
            n255 = Sine(x=w640) -> (sin(x)=w635:dbl)
            n256 = Equal?(x=w646, y=0) -> (x = y?=w630:bool)
            n257 = Multiply(x=w638, y=w639) -> (x*y=w637:dbl)
            n258 = Divide(x=w637, y=w636) -> (x/y=w633:dbl)
            n259 = case shown="False" w634 {
              tunnel: w650 -> [w700 _]
              tunnel: w647 -> [w699 _]
              tunnel: w633 -> [w698 _]
              tunnel: w632 -> [w695 _]
              tunnel: [w694 w701] -> w627
              frame False {
                n260 = Divide(x=w700, y=w699) -> (x/y=w697:dbl[])
                n261 = Multiply(x=w697, y=w698) -> (x*y=w696:dbl[])
                n262 = Add(x=w695, y=w696) -> (x+y=w694:dbl[])
              }
              frame True {
                w702 = 0.0
                n263 = Build Array(w702, w702) -> (w701:dbl[])
              }
            }
            n264 = Divide(x=w637, y=w635) -> (x/y=w600:dbl)
            n265 = case shown="False" w630 {
              tunnel: w649 -> [w691 _]
              tunnel: w646 -> [w685 _]
              tunnel: w600 -> [w690 _]
              tunnel: w629 -> [w686 _]
              tunnel: [w687 w692] -> w628
              tunnel: [w686 _] -> w599
              tunnel: [w685 _] -> w598
              frame False {
                n266 = Divide(x=w691, y=w685) -> (x/y=w689:dbl[])
                n267 = Multiply(x=w689, y=w690) -> (x*y=w688:dbl[])
                n268 = Add(x=w686, y=w688) -> (x+y=w687:dbl[])
              }
              frame True {
                w693 = 0.0
                n269 = Build Array(w693, w693) -> (w692:dbl[])
              }
            }
            n270 = call "IncenterTriangle.vi"("C"=w628, "B"=w627, "A"=w605, "Utilities in"=w602) -> ("I"=w615:dbl[])  [unwired: 5 in, 2 out]
            n271 = Subtract(x=w615, y=w623) -> (x-y=w624:dbl[])
            n272 = Negate(x=w623) -> (-x=w622:dbl[])
            n273 = call "AngleBetween2Vectors.vi"("Array 1"=w622, "Array 2"=w624, "Utilities in"=w602) -> ("Numeric"=w621:dbl)  [unwired: 6 in, 2 out]
            n274 = Less Or Equal?(x=w621, y=w625) -> (x <= y?=w616:bool)
            n275 = case shown="False" w616 {
              tunnel: w615 -> [_ w684]
              tunnel: [w668 w684] -> w614
              tunnel: w613 -> [w673 w683]
              tunnel: [w666 w683] -> w612
              tunnel: w611 -> [_ w682]
              tunnel: [w662 w682] -> w610
              tunnel: w609 -> [_ w681]
              tunnel: w608 -> [w664 w680]
              tunnel: [w665 w681] -> w607
              tunnel: [w664 w680] -> w606
              tunnel: w605 -> [w672 _]
              tunnel: w604 -> [w669 _]
              tunnel: w603 -> [w665 _]
              tunnel: w602 -> [w661 _]
              tunnel: w600 -> [w656 _]
              tunnel: w599 -> [w655 _]
              tunnel: w598 -> [w653 _]
              frame False {
                # "Tem que fazer isso pra colocar o ponto na posição correta e em relação ao centro do campo"
                # "Novo Gap"
                # "Se o os vetores estiverem abaixo do meio campo\npega o veotr pra baixo\nSe estiverem acima, pega o voter de cima"
                n276 = Index Array(array=w673) -> (element #1=w671:dbl[], element #2=w652:dbl[])  [unwired: 4 in]
                n277 = Index Array(array=w671) -> (element #2=w660:dbl)  [unwired: 2 in, 1 out]
                n278 = Greater?(x=w660, y=0.0) -> (0:w670:bool)
                n279 = Divide(x=w652, y=w653) -> (x/y=w658:dbl[])
                n280 = Multiply(x=w658, y=w656) -> (x*y=w657:dbl[])
                n281 = case shown="False" w670 {
                  tunnel: w669 -> [w678 w679]
                  tunnel: [w674 w679] -> w667
                  frame False {
                    # "Pega o vetor de baixo"
                    n282 = Index Array(array=w678) -> (element #1=w675:dbl, element #2=w677:dbl)  [unwired: 2 in]
                    n283 = Negate(x=w677) -> (-x=w676:dbl)
                    n284 = Build Array(w675, w676) -> (w674:dbl[])
                  }
                  frame True {
                  }
                }
                n285 = Add(x=w655, y=w657) -> (x+y=w654:dbl[])
                n286 = call "IncenterTriangle.vi"("C"=w654, "B"=w672, "A"=w667, "Utilities in"=w661) -> ("I"=w668:dbl[])  [unwired: 5 in, 2 out]
                n287 = Build Array(w667, w652) -> (w666:dbl[][])
                n288 = Subtract(x=w665, y=w664) -> (x-y=w663:dbl)
                n289 = Absolute Value(x=w663) -> (abs(x)=w662:dbl)
              }
              frame True {
              }
            }
            n290 = Bundle(w612, w610, "Numeric"=w607, "Numeric"=w606, "I"=w614) -> (w601:T3)  [unwired: 1 in]
          }
          n291 = for {
            tunnel: w407 -> [w530] mode=indexing
            shift-right: [w528] -> _
            shift-left: 10000.0 ("Numeric") -> [w527]
            shift-right: [w525] -> _
            shift-left: -10000.0 ("Numeric") -> [w524]
            shift-right: [w523] -> w413
            shift-left: dbl[] [] -> [w522]
            shift-right: [w520] -> w399
            shift-left: dbl[] [] -> [w519]
            shift-right: [w517] -> w418
            shift-left: 0.0 ("Numeric") -> [w516]
            shift-right: [w513] -> w404
            shift-left: 0.0 ("Numeric") -> [w512]
            # "Pegar aqui o maior y"
            # "Pegar aqui o menor y"
            n292 = Unbundle(w530) -> (w529:dbl[][], "Numeric"=w515:dbl)  [unwired: 3 out]
            n293 = Index Array(array=w529) -> (element #2=w521:dbl[])  [unwired: 4 in, 1 out]
            n294 = Index Array(array=w521) -> (element #2=w526:dbl)  [unwired: 2 in, 1 out]
            n295 = Less?(x=w526, y=w527) -> (x < y?=w518:bool)
            n296 = Greater?(x=w526, y=w524) -> (0:w514:bool)
            n297 = Select(t=w526, s=w518, f=w527) -> (s? t:f=w528:dbl)
            n298 = Select(t=w521, s=w518, f=w522) -> (s? t:f=w523:dbl[])
            n299 = Select(t=w515, s=w518, f=w516) -> (s? t:f=w517:dbl)
            n300 = Select(t=w515, s=w514, f=w512) -> (s? t:f=w513:dbl)
            n301 = Select(t=w521, s=w514, f=w519) -> (s? t:f=w520:dbl[])
            n302 = Select(t=w526, s=w514, f=w524) -> (s? t:f=w525:dbl)
          }
          n303 = Index Array(array=w394) -> (element #1=w421:dbl, element #2=w423:dbl)  [unwired: 2 in]
          n304 = Negate(x=w423) -> (-x=w422:dbl)
          n305 = Build Array(w421, w422) -> (w409:dbl[])
          n306 = Add(x=w403, y=w418) -> (x+y=w417:dbl)
          n307 = Add(x=w403, y=w404) -> (x+y=w402:dbl)
          n308 = call-dynamic "Module.vi"("2D vector"=w399, "Utilities in"=w384) -> ("Modulo"=w398:dbl)  [unwired: 7 in, 2 out]
          n309 = call-dynamic "Module.vi"("2D vector"=w413, "Utilities in"=w385) -> ("Modulo"=w412:dbl)  [unwired: 7 in, 2 out]
          n310 = Sine(x=w403) -> (sin(x)=w415:dbl)
          n311 = Sine(x=w402) -> (sin(x)=w401:dbl)
          n312 = Sine(x=w417) -> (sin(x)=w414:dbl)
          n313 = call "AngleBetween2Vectors.vi"("Array 1"=w399, "Array 2"=w394, "Utilities in"=w384) -> ("Numeric"=w386:dbl)  [unwired: 6 in, 2 out]
          n314 = Equal?(x=w412, y=0) -> (x = y?=w419:bool)
          n315 = call "AngleBetween2Vectors.vi"("Array 1"=w413, "Array 2"=w409, "Utilities in"=w385) -> ("Numeric"=w389:dbl)  [unwired: 6 in, 2 out]
          n316 = Multiply(x=w416, y=w415) -> (x*y=w400:dbl)
          n317 = Divide(x=w400, y=w401) -> (x/y=w397:dbl)
          n318 = Equal?(x=w398, y=0) -> (x = y?=w405:bool)
          n319 = Divide(x=w400, y=w414) -> (x/y=w411:dbl)
          n320 = case shown="False" w419 {
            tunnel: w413 -> [w509 _]
            tunnel: w412 -> [w508 _]
            tunnel: w411 -> [w507 _]
            tunnel: w395 -> [w504 _]
            tunnel: [w503 w510] -> w410
            frame False {
              n321 = Divide(x=w509, y=w508) -> (x/y=w506:dbl[])
              n322 = Multiply(x=w506, y=w507) -> (x*y=w505:dbl[])
              n323 = Add(x=w504, y=w505) -> (x+y=w503:dbl[])
            }
            frame True {
              w511 = 0.0
              n324 = Build Array(w511, w511) -> (w510:dbl[])
            }
          }
          n325 = case shown="False" w405 {
            tunnel: w398 -> [w500 _]
            tunnel: w399 -> [w499 _]
            tunnel: w397 -> [w498 _]
            tunnel: w395 -> [w495 _]
            tunnel: [w494 w501] -> w396
            frame False {
              n326 = Divide(x=w500, y=w499) -> (x/y=w497:dbl[])
              n327 = Multiply(x=w497, y=w498) -> (x*y=w496:dbl[])
              n328 = Add(x=w495, y=w496) -> (x+y=w494:dbl[])
            }
            frame True {
              w502 = 0.0
              n329 = Build Array(w502, w502) -> (w501:dbl[])
            }
          }
          n330 = Add(x=w409, y=w395) -> (x+y=w408:dbl[])
          n331 = Add(x=w395, y=w394) -> (x+y=w393:dbl[])
          n332 = call "IncenterTriangle.vi"("C"=w395, "B"=w410, "A"=w408, "Utilities in"=w385) -> ("I"=w391:dbl[])  [unwired: 5 in, 2 out]
          n333 = call "IncenterTriangle.vi"("C"=w393, "B"=w395, "A"=w396, "Utilities in"=w385) -> ("I"=w387:dbl[])  [unwired: 5 in, 2 out]
          n334 = Greater?(x=w389, y=w386) -> (0:w392:bool)
          n335 = case shown="False" w392 {
            tunnel: w391 -> [_ w493]
            tunnel: [w491 w493] -> w390
            tunnel: w389 -> [_ w492]
            tunnel: [w490 w492] -> w388
            tunnel: w387 -> [w491 _]
            tunnel: w386 -> [w490 _]
            frame False {
            }
            frame True {
            }
          }
          n336 = for {
            tunnel: w407 -> [w541] mode=indexing
            shift-right: [w540] -> _
            shift-left: w388 -> [w534]
            shift-right: [w538] -> w437
            shift-left: w390 -> [w537]
            # "Vai retornar o incentro"
            n337 = Unbundle(w541) -> (w535:dbl, "I"=w539:dbl[])  [unwired: 3 out]
            n338 = Less?(x=w534, y=w535) -> (x < y?=w536:bool)
            n339 = Select(t=w539, s=w536, f=w537) -> (s? t:f=w538:dbl[])
            n340 = Select(t=w535, s=w536, f=w534) -> (s? t:f=w540:dbl)
          }
          n341 = call "FindRobotByRole.vi"("role"=roles."PreparePassReceiver", "RobotRef"=w463, "Utilities in"=w464) -> ("Robots"=w461:refnum<class "Robot.lvclass">[])  [unwired: 6 in, 2 out]
          n342 = property class="Robot"(reference=w460) -> ("id"=w459:i32)  [unwired: 1 in, 2 out]
          n343 = for {
            tunnel: w461 -> [w565] mode=indexing
            tunnel: w459 -> [w566]
            tunnel: [w562] -> w458 mode=indexing if=w561
            n344 = property class="Robot"(reference=w565) -> ("id"=w567:i32, "x"=w564:dbl, "y"=w563:dbl)  [unwired: 1 in, 2 out]
            n345 = Not Equal?(x=w567, y=w566) -> (x != y?=w561:bool)
            n346 = Build Array(w564, w563) -> (w562:dbl[])
          }
          n347 = Index Array(array=w458) -> (element=w457:dbl[])  [unwired: 2 in]
          n348 = call-dynamic "Distance.vi"("P1"=w437, "P2"=w457, "Utilities in"=w464) -> ("Distance"=w456:dbl)  [unwired: 6 in, 2 out]
          n349 = Divide(x=w449, y=3.0) -> (x/y=w447:dbl)
          n350 = Less?(x=w456, y=w447) -> (x < y?=w455:bool)
          n351 = case shown="True" w455 {
            tunnel: [w568 w570] -> w436
            tunnel: w437 -> [w568 w569]
            frame False {
              # "Se der falso, pasa a posição calculada anteriormente"
            }
            frame True {
              # "se der true, ele se move em direção ao centro do campo"
              n352 = Multiply(x=w569, y=0.6) -> (x*y=w570:dbl[])
            }
          }
          n353 = property class="Ball"(reference=w478) -> ("x"=w477:dbl, "y"=w454:dbl)  [unwired: 1 in, 2 out]
          n354 = Build Array(w477, w454) -> (w473:dbl[])
          n355 = call-dynamic "DistancePointLine.vi"("Q"=w436, "P2"=w473, "P1"=w395, "Utilities in"=w464) -> ("distance"=w476:dbl)  [unwired: 5 in, 2 out]
          n356 = Less Or Equal?(x=w476, y=200.0) -> (x <= y?=w435:bool)
          n357 = case shown="True" w435 {
            tunnel: [w572 w580] -> w474
            tunnel: w473 -> [_ w588]
            tunnel: w395 -> [_ w587]
            tunnel: w454 -> [_ w576]
            tunnel: w436 -> [w572 w573]
            frame False {
            }
            frame True {
              # "Se ybola>0, pega o vetor (-b,a) caso contrario, pega o (b,-a)"
              # "Soma com o vetor x pra fazer em relação ao centro do  campo"
              # "normaliza ele"
              # "(a,b) o perpendicular em direção\n ao entro do campo é (-b,a)\nbola na parte de cima"
              # "Vetor bola-gol"
              # "Ele se move na perpendicular em relação à reta bola gol\nem direção ao meio do campo"
              # "Distância do robo ate a linha da bola-gol"
              n358 = Subtract(x=w588, y=w587) -> (x-y=w586:dbl[])
              n359 = Index Array(array=w586) -> (element #1=w578:dbl, element #2=w579:dbl)  [unwired: 2 in]
              n360 = Greater?(x=w576, y=0.0) -> (0:w574:bool)
              n361 = case shown="False" w574 {
                tunnel: w579 -> [w592 w593]
                tunnel: w578 -> [w590 w595]
                tunnel: [w589 w596] -> w577
                frame True {
                  n362 = Negate(x=w592) -> (-x=w591:dbl)
                  n363 = Build Array(w591, w590) -> (w589:dbl[])
                }
                frame False {
                  n364 = Negate(x=w595) -> (-x=w594:dbl)
                  n365 = Build Array(w593, w594) -> (w596:dbl[])
                }
              }
              n366 = call-dynamic "Module.vi"("2D vector"=w577, "Utilities in"=refnum<class "Utilities.lvclass"> refnum) -> ("Modulo"=w584:dbl)  [unwired: 7 in, 2 out]
              n367 = Divide(x=w577, y=w584) -> (x/y=w583:dbl[])
              n368 = Multiply(x=600.0, y=w583) -> (x*y=w581:dbl[])
              n369 = Add(x=w573, y=w581) -> (x+y=w580:dbl[])
            }
          }
        }
      }
    }
    frame Error {
    }
  }
  "error out" <- w13
  "2ndStrikerPositionSkill out" <- w14
  "2nd Striker Position" <- w6
